vi "GUI_Cameras_GRID.vi"() -> ()   [LabVIEW 2011]
uses:
  <vilib>/Utility/miscctls.llb/LVRectTypeDef.ctl
  <vilib>/vision/NI_Vision_Development_Module.lvlib
panel:
  in  "Tab Control":T1(tab)
  in  "analysis":bool
  out "MaxCounts":dbl(slide) scale=0.0..256.0
  in  "triggerdelay":dbl
  in  "trigger":bool
  in  "save":bool
  in  "exposure":dbl=0.52 caption="Exposure"
  in  "gain":dbl
  in  "shotnumber":i32=354
  out "Centroid":cluster{"X Centroid":sgl, "Y Centroid":sgl} {"Y Centroid" format="%.2f"; "X Centroid" format="%.2f"}
  out "Mean Value":sgl format="%.2f"
  out "Mean Value 2":sgl(graph)
  out "histogram":T2(graph)
  out "lineout":cluster{"x0":sgl, "dx":sgl, "Pixels Line":sgl[]}(graph)
  out "analysis error":errorcluster
  out "Zoom changed":bool
  out "Zoom old":cluster{"X":sgl, "Y":sgl}
  out "ratio(h)":bool=TRUE
  out "fixsize":bool
  out "Change Ratio":cluster{"X":sgl, "Y":sgl}={"X"=1.6671598, "Y"=0.6151203}
  out "old Panel Bounds":T3={"Left"=105, "Top"=80, "Right"=781, "Bottom"=662}
  out "error (h)":bool
  in  "Main Tap":enum32{"IMAQ", "Network", "Internal", "Array"}(tab)
  out "Image (IMAQ)":T4(plugin-control)
  out "local Port":u16=65401
  out "Remote Host":string="192.168.10.157"
  out "port or service name":u16=65400
  in  "timeout ms (slow resp)":i32=500
  in  "reset":bool
  out "All Devices (h)":string[](array[string])
  out "centroidy":dbl
  out "fast ID (h)":refnum<k16>
  out "slow ID (h)":refnum<k16>
  out "error out":errorcluster
  out "connections (hidden)":variant[](array[variant])=[variant(refnum<k16> refnum), variant(refnum<k16> refnum)]
  in  "time to wait (main loop)":i32=200
  in  "time to wait (TCP)":i32=10
  out "Data String":string="exposure,0.520000\r\ntrigger,off\r\nsave,off\r\ngain,0.000000\r\n"
  in  "send":bool
  in  "localsavingpath":path
  out "centroidy":dbl
  out "Image (array)":u8[][](graph)
  out "Device Name (h)":string="FakeCam1"
  out "stop":bool
  out "error message":string
  out "image connection":bool
  out "data connection ok":bool
  # "Data"
  # "Image"
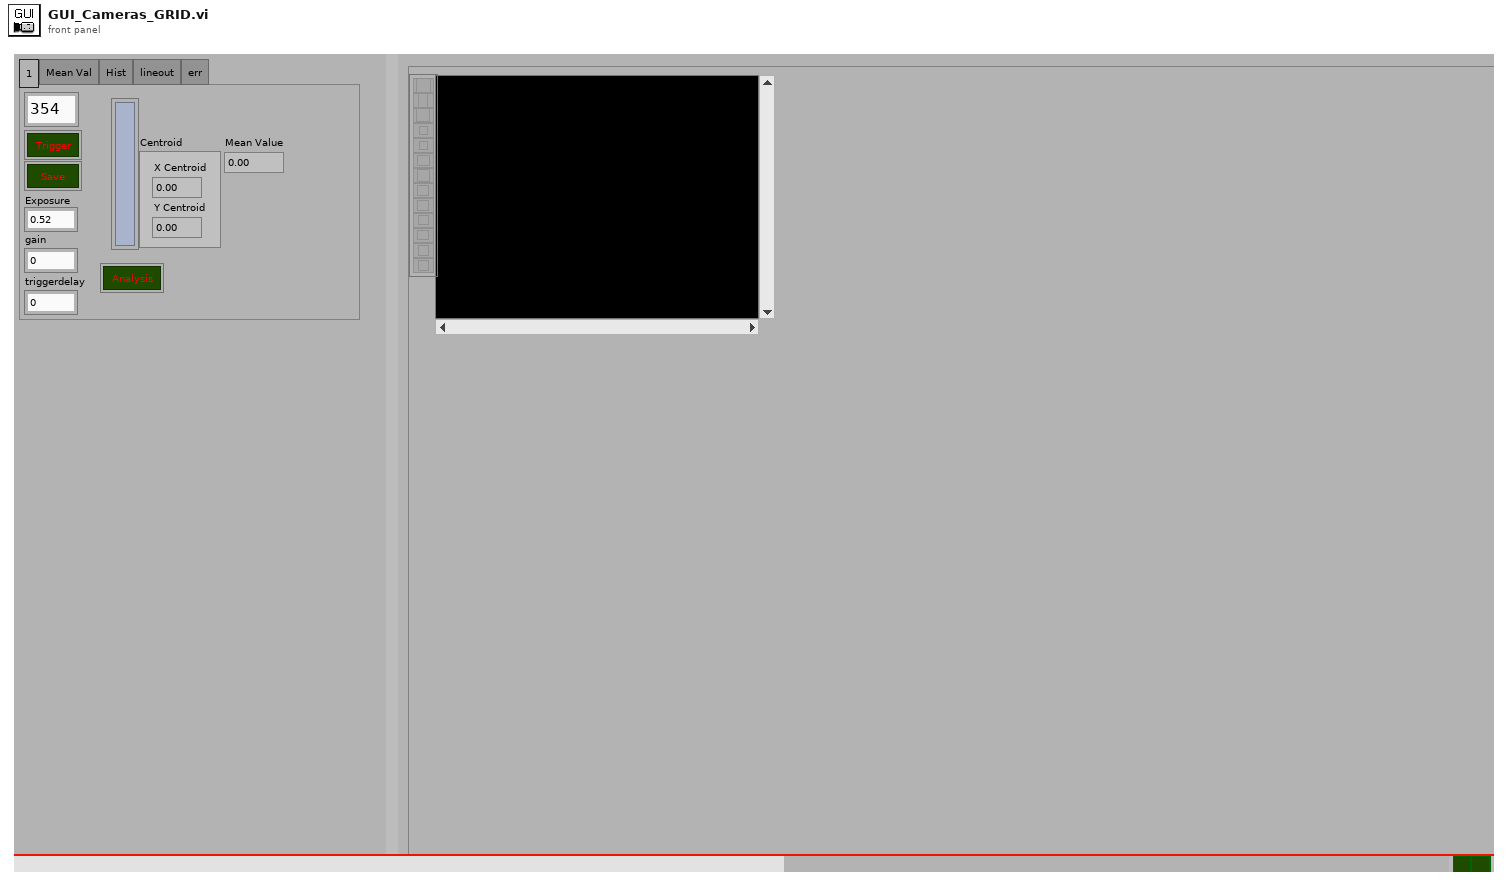
[diagram p1: front panel]
types:
  T1 = enum32{"1", "Mean Val", "Hist", "lineout", "err"}
  T2 = cluster{"Starting Value":sgl, "Incremental Value":sgl, "Histogram":u32[]}
  T3 = typedef "LVRectTypeDef.ctl" = cluster{"Left":i16, "Top":i16, "Right":i16, "Bottom":i16}
  T4 = typedef "IMAQ Image.ctl" = refnum<image>
  T5 = enum16{"Grayscale", "Binary", "Gradient", "Rainbow", "Temperature", "User Defined"}
  T6 = typedef "Image Type" = u32
  T7 = cluster{"Global Rectangle":i32[], "Contours":cluster{"Contour Type":u32, "ROI Type":u32, "Points":i32[]}[]}
  T8 = typedef "IMAQ Line" = cluster{"Start X":i32, "Start Y":i32, "End X":i32, "End Y":i32}
  T9 = typedef "ROI Descriptor" = cluster{"Global Rectangle":i32[], "Contours":cluster{"ID":enum32{"External", "Internal"}, "Type":u32, "Coordinates":i32[]}[]}
  T10 = typedef "LVBoundsTypeDef.ctl" = cluster{"Width":u32, "Height":u32}
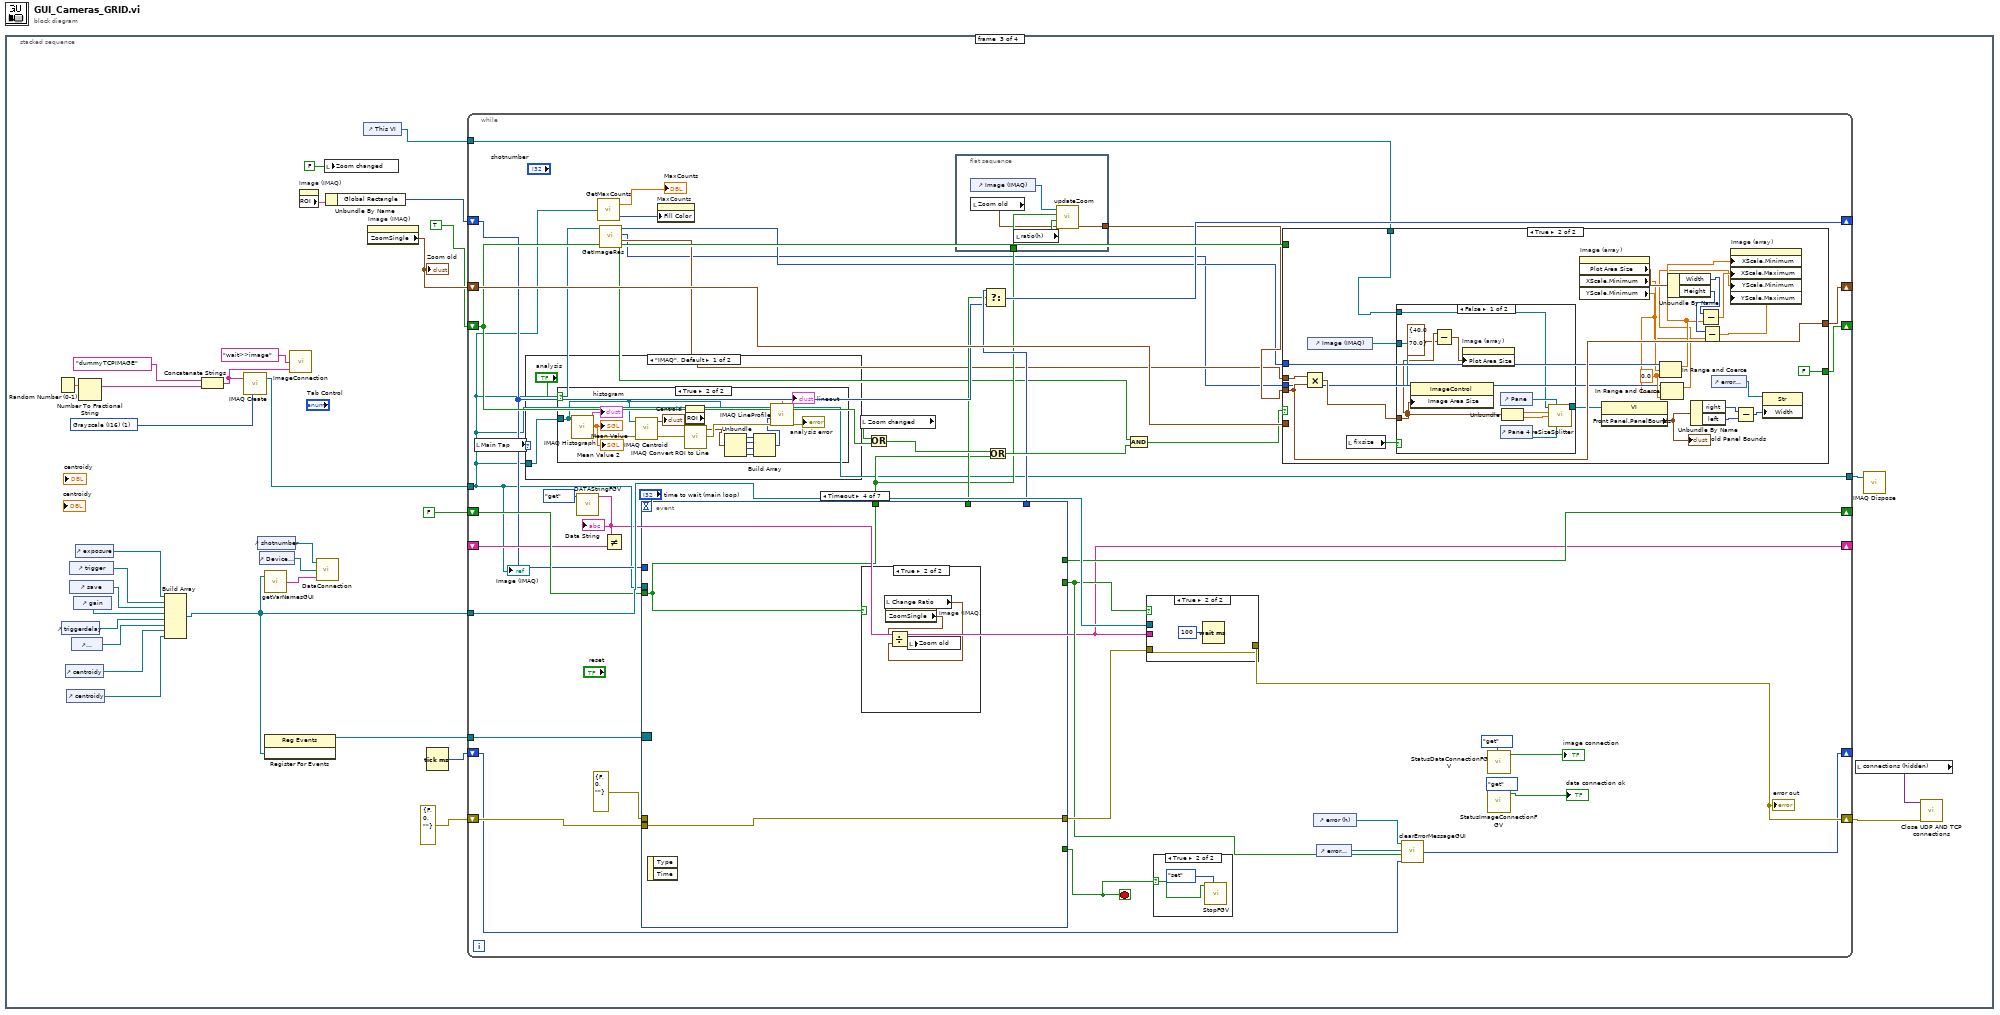
[diagram p0: block diagram]
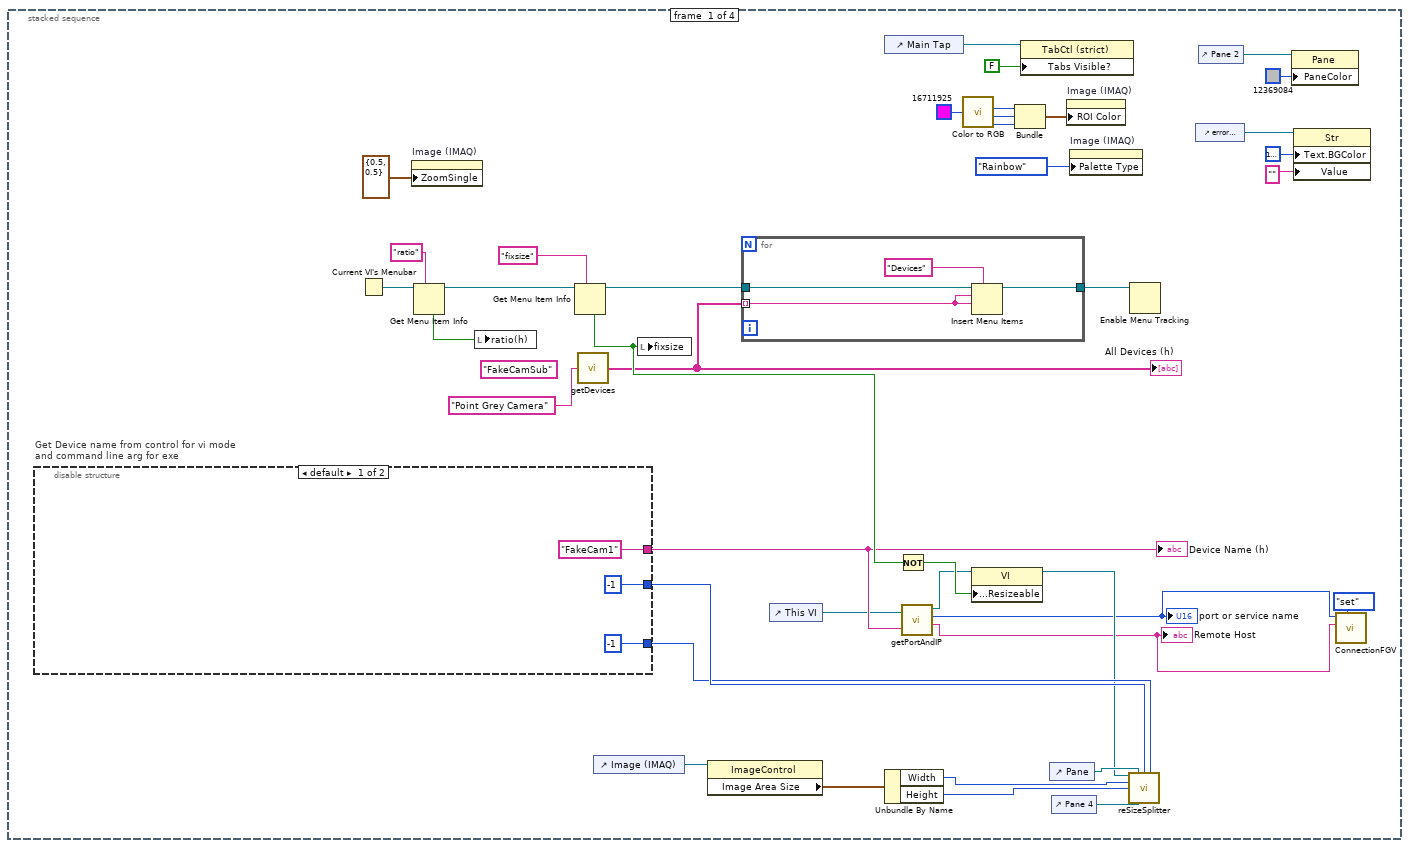
[diagram p2: hidden frame]
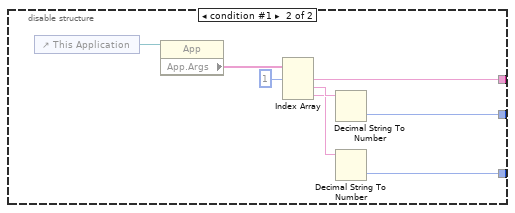
[diagram p3: hidden frame]
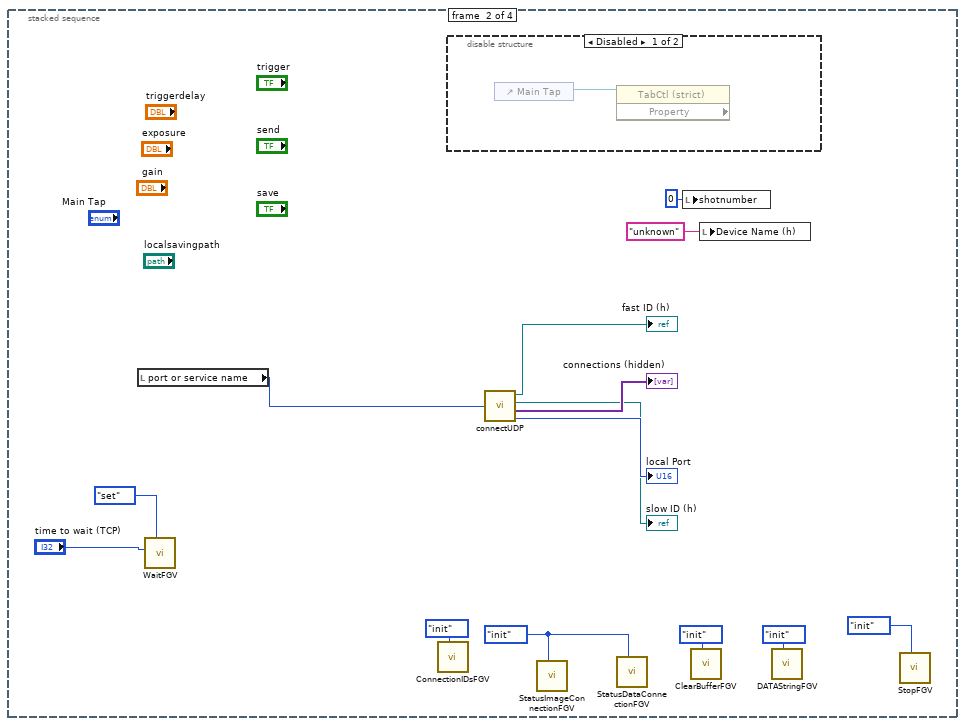
[diagram p4: hidden frame]
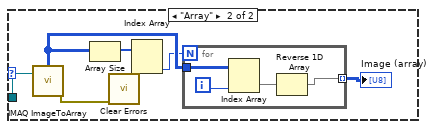
[diagram p8: hidden frame]
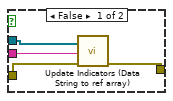
[diagram p11: hidden frame]
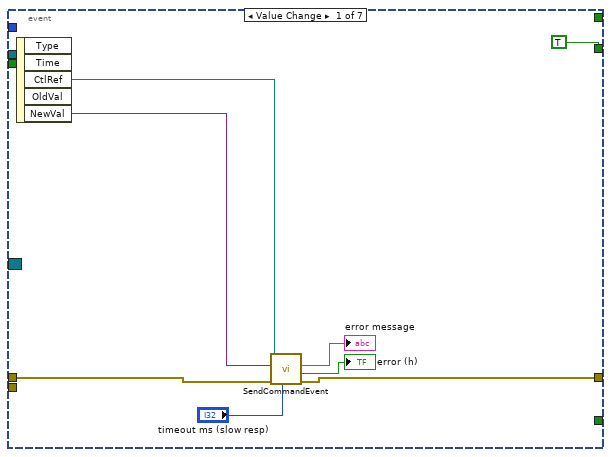
[diagram p12: hidden frame]
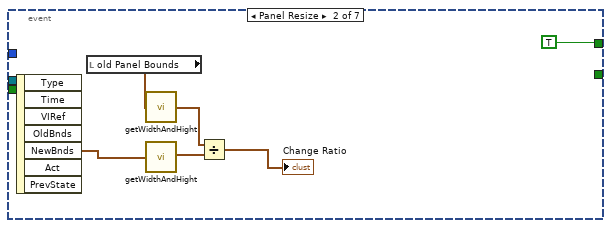
[diagram p13: hidden frame]
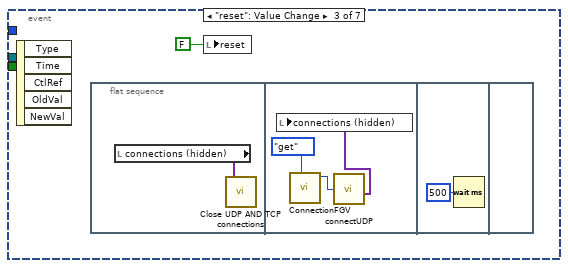
[diagram p14: hidden frame]
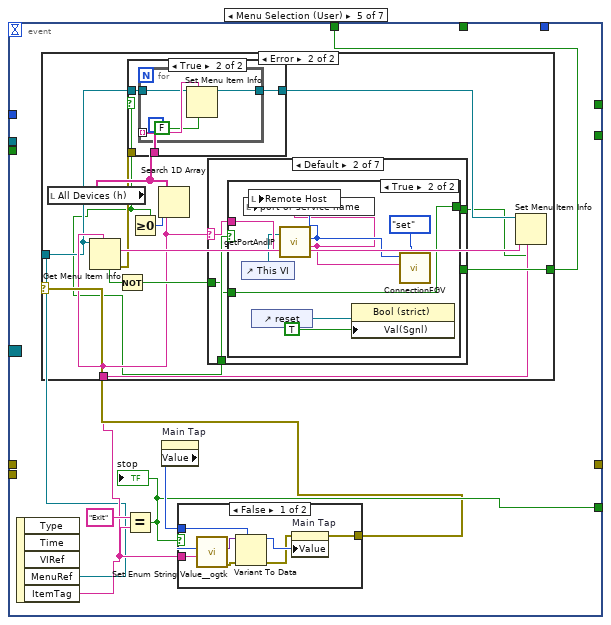
[diagram p16: hidden frame]
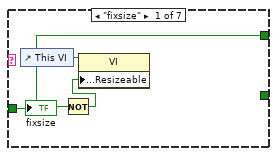
[diagram p19: hidden frame]
diagram:
  n1 = stacked-sequence {
    frame #0 {
      (unwired) "FakeCamSub" ("Device Class")
      n2 = disable-structure "Get Device name from control for vi mode\nand command line arg for exe" shown="default" {
        disable-tunnel: ["FakeCam1" ("Device Name for vi mode") w52] -> w14
        disable-tunnel: [i16 -1 ("left") w49] -> w27
        disable-tunnel: [i16 -1 ("left") w48] -> w26
        frame condition #0 (active) {
        }
        frame condition #1 {
          n3 = control-ref of="This Application"() -> (w55:refnum<vi>)
          n4 = property class="App"(reference=w55) -> ("App.Args"=w54:string[])  [unwired: 1 in, 2 out]
          n5 = Index Array(array=w54, index #1=1 ("index")) -> (element #1=w52:string, element #2=w51:string, element #3=w50:string)  [unwired: 2 in]
          n6 = Decimal String To Number(string=w51) -> (number=w49:i32)  [unwired: 2 in, 1 out]
          n7 = Decimal String To Number(string=w50) -> (number=w48:i32)  [unwired: 2 in, 1 out]
        }
      }
      "Device Name (h)" <- w14
      n8 = Current VI's Menubar() -> (w31:refnum<k9>)
      n9 = property on="Image (IMAQ)" class="ImageControl"("ZoomSingle"=cluster{"X":sgl, "Y":sgl} {"X"=0.5, "Y"=0.5} ("ZoomSingle:All Elements")) -> ()  [unwired: 2 in, 2 out]
      n10 = Get Menu Item Info(7:"ratio" ("item tag"), 11:w31) -> (3:w29:refnum<k9>, 4:w30:bool)  [unwired: 1 in, 5 out]
      n11 = local write "ratio(h)"(w30) -> ()
      n12 = Get Menu Item Info(7:"fixsize" ("item tag"), 11:w29) -> (3:w17:refnum<k9>, 4:w24:bool)  [unwired: 1 in, 5 out]
      n13 = call "getDevices.vi"("Device Class"="Point Grey Camera") -> ("All Devices"=w15:string[])
      "All Devices (h)" <- w15
      n14 = control-ref of="Image (IMAQ)"() -> (w38:refnum<vi>)
      n15 = local write "fixsize"(w24) -> ()
      n16 = property class="ImageControl"(reference=w38) -> ("Image Area Size"=w37:cluster{"Width":u32, "Height":u32})  [unwired: 1 in, 2 out]
      n17 = for {
        tunnel: w17 -> [w44]
        tunnel: [w43] -> w16
        tunnel: w15 -> [w41] mode=indexing
        n18 = Insert Menu Items(5:"Devices" ("menu tag"), 7:w41, 8:w41, 9:w44) -> (3:w43:refnum<k9>)  [unwired: 2 in, 2 out]
      }
      n19 = control-ref of="This VI"() -> (w13:refnum<vi>)
      n20 = control-ref of="Main Tap"() -> (w40:refnum<vi>)
      n21 = Unbundle By Name(w37) -> ("Width"=w36:u32, "Height"=w35:u32)
      n22 = Not(x=w24) -> (.not. x?=w25:bool)
      n23 = call "getPortAndIP.vi"("This Vi"=w13, "Device Name"=w14) -> ("reference out"=w12:refnum<vi>, "port or service name"=w3:u16, "Remote Host"=w2:string)  [unwired: 1 in]
      "port or service name" <- w3
      "Remote Host" <- w2
      n24 = call <vilib>:"Color to RGB.vi"("Color"=u32 16711925) -> ("R"=w9:u8, "G"=w8:u8, "B"=w7:u8)  [unwired: 1 out]
      n25 = property class="VI"(reference=w12, "Front Panel.Resizeable"=w25) -> (reference out=w5:refnum<vi>)  [unwired: 1 in, 1 out]
      n26 = Bundle("R"=w9, "G"=w8, "B"=w7) -> (w6:cluster{"R":u8, "G":u8, "B":u8})  [unwired: 1 in]
      n27 = property class="TabCtl (strict)"(reference=w40, "Tabs Visible?"=FALSE) -> ()  [unwired: 1 in, 2 out]
      n28 = control-ref of="Pane"() -> (w34:refnum<vi>)
      n29 = control-ref of="Pane 4"() -> (w23:refnum<vi>)
      n30 = property on="Image (IMAQ)" class="ImageControl"("ROI Color"=w6) -> ()  [unwired: 2 in, 2 out]
      n31 = property on="Image (IMAQ)" class="ImageControl"("Palette Type"=T5."Rainbow" ("Palette:Palette Type")) -> ()  [unwired: 2 in, 2 out]
      n32 = call "reSizeSplitter.vi"("this vi"=w5, "pane"=w34, "left"=w27, "top"=w26, "Width"=w36, "Height"=w35, "pane2"=w23) -> ()  [unwired: 8 in, 1 out]
      n33 = Enable Menu Tracking(4:w16) -> ()  [unwired: 2 in, 2 out]
      n34 = control-ref of="error message"() -> (w21:refnum<vi>)
      n35 = control-ref of="Pane 2"() -> (w19:refnum<vi>)
      n36 = property class="Pane"(reference=w19, "PaneColor"=u32 12369084) -> ()  [unwired: 1 in, 2 out]
      n37 = property class="Str"(reference=w21, "Text.BGColor"=u32 16777238, "Value"="") -> ()  [unwired: 1 in, 2 out]
      n38 = call "ConnectionFGV.vi"("command"=enum16{"get", "set", "init"}."set", "Remote Host in"=w2, "port or service name in"=w3) -> ()  [unwired: 7 in, 2 out]
    }
    frame #1 {
      w65 = enum16{"get", "set", "init"}."init" ("Command")
      n39 = local read "port or service name"() -> (w67:u16)
      n40 = call "WaitFGV.vi"("Command"=enum16{"get", "set", "init"}."set", "milliseconds to wait"="time to wait (TCP)") -> ()  [unwired: 9 in, 1 out]
      n41 = call "ConnectionIDsFGV.vi"("Command"=enum16{"add", "get", "init"}."init") -> ()  [unwired: 10 in, 1 out]
      n42 = disable-structure shown="Disabled" {
        frame Disabled {
          n43 = control-ref of="Main Tap"() -> (w70:refnum<vi>)
          n44 = property class="TabCtl (strict)" props=[](reference=w70) -> ()  [unwired: 1 in, 3 out]
        }
        frame Enabled {
        }
      }
      n45 = call "connectUDP.vi"("port or service name"=w67) -> ("fast ID (h)"=→"fast ID (h)":refnum<k16>, "slow ID (h)"=→"slow ID (h)":refnum<k16>, "connections (hidden)"=→"connections (hidden)":variant[], "local Port"=→"local Port":u16)
      n46 = call "StatusImageConnectionFGV.vi"("Command"=w65) -> ()  [unwired: 10 in, 1 out]
      n47 = call "StatusDataConnectionFGV.vi"("Command"=w65) -> ()  [unwired: 10 in, 1 out]
      n48 = local write "shotnumber"(0 ("shotnumber")) -> ()
      n49 = call "ClearBufferFGV.vi"("Command"=enum16{"set", "get", "init"}."init") -> ()  [unwired: 10 in, 1 out]
      n50 = local write "Device Name (h)"("unknown" ("Device Name")) -> ()
      n51 = call "DATAStringFGV.vi"("Command"=enum16{"get", "set", "init"}."init") -> ()  [unwired: 10 in, 1 out]
      n52 = call "StopFGV.vi"("Command"=enum16{"set", "get", "init"}."init") -> ()  [unwired: 10 in, 1 out]
    }
    frame #2 {
      w100 = T6 1 items=["Grayscale (U8)", "Grayscale (I16)", "Grayscale (SGL)", "Complex (CSG)", "RGB (U32)", "HSL (U32)", "RGB (U64)", "Grayscale (U16)"] ("Image Type")
      n53 = Random Number (0-1)() -> (number: 0 to 1=w97:dbl)
      n54 = control-ref of="triggerdelay"() -> (w87:refnum<vi>)
      n55 = control-ref of="centroidy"() -> (w81:refnum<vi>)
      n56 = control-ref of="centroidy"() -> (w74:refnum<vi>)
      n57 = control-ref of="trigger"() -> (w91:refnum<vi>)
      n58 = control-ref of="save"() -> (w89:refnum<vi>)
      n59 = control-ref of="localsavingpath"() -> (w82:refnum<vi>)
      n60 = control-ref of="gain"() -> (w88:refnum<vi>)
      n61 = control-ref of="exposure"() -> (w90:refnum<vi>)
      n62 = Number To Fractional String(number=w97) -> (F-format string=w96:string)  [unwired: 3 in]
      n63 = Build Array(w90, w91, w89, w88, w87, w82, w81, w74) -> (w72:refnum<vi>[])
      n64 = Concatenate Strings("dummyTCPIMAGE" ("Image Name"), w96) -> (w94:string)
      n65 = call "IMAQ Create"("Image Name"=w94, "Image Type"=w100) -> ("New Image"=w99:T4)  [unwired: 3 in, 1 out]
      n66 = control-ref of="shotnumber"() -> (w76:refnum<vi>)
      n67 = control-ref of="Device Name (h)"() -> (w75:refnum<vi>)
      n68 = call "getVarNamesGUI.vi"("Array"=w72) -> ("String"=w71:string)  [unwired: 1 in]
      n69 = register-events(w72) -> (reference out=w73:refnum<event-registration>)  [unwired: 2 in, 1 out]
      n70 = call "ImageConnection.vi"("Image Name"=w94, "Image Subscriber list"="wait>>image") -> ()  [unwired: 2 in]
      n71 = property on="Image (IMAQ)" class="ImageControl"() -> ("ROI"=w80:T7)  [unwired: 2 in, 2 out]
      n72 = call "DataConnection.vi"("Subscriber list"=w71, "Device Name (h)"=w75, "shotnumber"=w76) -> ()
      n73 = local write "Zoom changed"(FALSE ("Zoom changed")) -> ()
      n74 = Unbundle By Name(w80) -> ("Global Rectangle"=w79:i32[])
      n75 = control-ref of="This VI"() -> (w78:refnum<vi>)
      n76 = property on="Image (IMAQ)" class="ImageControl"() -> ("ZoomSingle"=w86:cluster{"X":sgl, "Y":sgl})  [unwired: 2 in, 2 out]
      "Zoom old" <- w86
      n77 = Tick Count (ms)() -> (millisecond timer value=w83:u32)
      n78 = while {
        shift-right: [w142] -> w98
        shift-left: errorcluster {"status"=FALSE, "code"=0, "source"=""} ("error out") -> [w144]
        tunnel: w99 -> [w116]
        tunnel: [w116] -> w101
        tunnel: w72 -> [w146]
        shift-right: [w141] -> _
        shift-left: w86 -> [w140]
        shift-right: [w138] -> _
        shift-left: FALSE -> [w139]
        shift-right: [w137] -> _
        shift-left: TRUE -> [w136]
        shift-right: [w132] -> _
        shift-left: w83 -> [w131]
        shift-right: [w105] -> _
        shift-left: _ -> [w129]
        shift-right: [w125] -> _
        shift-left: w79 -> [w124]
        tunnel: w78 -> [w122]
        tunnel: w73 -> [w103]
        stop <- w106 stop-if-true
        n79 = local read "Main Tap"() -> (w127:enum32{"IMAQ", "Network", "Internal", "Array"})
        n80 = case shown="\"IMAQ\", Default" w127 {
          tunnel: w116 -> [w156 w177]
          frame "IMAQ", Default {
            n81 = case shown="True" "analysis" {
              tunnel: w156 -> [_ w167]
              frame False {
              }
              frame True {
                n82 = call "IMAQ Histograph"("Image"=w167) -> ("error out"=w169:errorcluster, "Mean Value"=→"Mean Value" →"Mean Value 2":sgl, "Histogram Graph"=→"histogram":T2)  [unwired: 7 in, 1 out]
                n83 = call "IMAQ Centroid"("error in (no error)"=w169, "Image"=w167) -> ("error out"=w166:errorcluster, "Centroid"=→"Centroid":cluster{"X Centroid":sgl, "Y Centroid":sgl})  [unwired: 2 in]
                n84 = property on="Image (IMAQ)" class="ImageControl"() -> ("ROI"=w163:T7)  [unwired: 2 in, 2 out]
                n85 = call "IMAQ Convert ROI to Line"("ROI Descriptor"=w163) -> ("Line"=w162:T8)  [unwired: 8 in, 1 out]
                n86 = Unbundle(w162) -> ("Start X"=w161:i32, "Start Y"=w160:i32, "End X"=w159:i32, "End Y"=w158:i32)
                n87 = Build Array(w161, w160, w159, w158) -> (w157:i32[])
                n88 = call "IMAQ LineProfile"("error in (no error)"=w166, "Line Coordinates"=w157, "Image"=w167) -> ("error out"=→"analysis error":errorcluster, "Line Graph"=→"lineout":cluster{"x0":sgl, "dx":sgl, "Pixels Line":sgl[]})  [unwired: 2 in, 2 out]
              }
            }
          }
          frame "Array" {
            n89 = call "IMAQ ImageToArray"("Image"=w177) -> ("error out"=w176:errorcluster, "Image Pixels (U8)"=w173:u8[][])  [unwired: 3 in, 3 out]
            n90 = Array Size(array=w173) -> (size(s)=w175:i32[])
            n91 = call <vilib>:"Clear Errors.vi"("error in (no error)"=w176) -> ()  [unwired: 6 in, 1 out]
            n92 = Index Array(array=w175) -> (element #2=w172:i32)  [unwired: 2 in, 1 out]
            n93 = for {
              N: w172 -> [_]
              tunnel: w173 -> [w181]
              tunnel: [w179] -> w174 mode=indexing
              i -> [w178]
              n94 = Index Array(array=w181, index (col)=w178) -> (element=w180:u8[])  [unwired: 1 in]
              n95 = Reverse 1D Array(array=w180) -> (reversed array=w179:u8[])
            }
            "Image (array)" <- w174
          }
        }
        n96 = call "DATAStringFGV.vi"("Command"=enum16{"get", "set", "init"}."get") -> ("Data String out"=w105:string)  [unwired: 10 in]
        "Data String" <- w105
        n97 = call "GetMaxCounts.vi"("New Image"=w116) -> ("Maximal Value"=→"MaxCounts":sgl, "Color"=w118:u32)
        n98 = call "GetImageRes.vi"("Image"=w116) -> ("valid Image"=w114:bool, "Image Area:Size:All Elements"=w115:cluster{"Width":u32, "Height":u32}, "Y Resolution"=w112:i32, "X Resolution"=w113:i32)  [unwired: 7 in]
        n99 = Not Equal?(x=w105, y=w129) -> ()  [unwired: 1 out]
        n100 = event shown="[3] Timeout" {
          selector: w103 -> [_ _ _ _ _ _ _]
          dyn-events: _ -> [_ _ _ _ _ _ _]
          timeout: "time to wait (main loop)" -> [_ _ _ _ _ _ _]
          tunnel: [w231 _ _ w247 _ _ _] -> w143
          tunnel: errorcluster {"status"=FALSE, "code"=0, "source"=""} ("error out") -> [w233 _ _ _ _ _ _]
          tunnel: w144 -> [_ _ _ w247 _ _ _]
          tunnel: [TRUE _ _ _ _ _ _] -> w128
          tunnel: [_ _ _ _ w255 _ _] -> w106
          tunnel: [_ _ _ w246 w252 _ _] -> w121
          tunnel: w139 -> [_ _ _ w246 _ _ _]
          tunnel: [_ TRUE _ _ _ _ _] -> w138
          tunnel: [_ _ _ _ _ _ w333] -> w126
          tunnel: w124 -> [_ _ _ _ _ _ w334]
          tunnel: [_ _ _ _ _ _ w327] -> w123
          tunnel: w116 -> [_ _ _ _ _ _ w336]
          event Value Change {
            n101 = event-data() -> ("CtlRef"=w228:refnum<vi>, "NewVal"=w227:variant)  [unwired: 1 in, 3 out]
            n102 = call "SendCommandEvent.vi"("timeout ms (slow resp)"="timeout ms (slow resp)", "error out 2"=w233, "NewVal"=w227, "CtlRef"=w228) -> ("error out"=w231:errorcluster, "error (h)"=→"error (h)":bool, "error message"=→"error message":string)  [unwired: 4 in, 1 out]
          }
          event Panel Resize {
            n103 = event-data() -> ("NewBnds"=w239:T3)  [unwired: 1 in, 6 out]
            n104 = local read "old Panel Bounds"() -> (w237:T3)
            n105 = call "getWidthAndHight.vi"("OldBnds"=w237) -> ("output cluster"=w236:cluster{"X":sgl, "Y":sgl})
            n106 = call "getWidthAndHight.vi"("OldBnds"=w239) -> ("output cluster"=w235:cluster{"X":sgl, "Y":sgl})
            n107 = Divide(x=w236, y=w235) -> (x/y=→"Change Ratio":cluster{"X":sgl, "Y":sgl})
          }
          event "reset": Value Change {
            n108 = event-data() -> ()  [unwired: 1 in, 5 out]
            n109 = flat-sequence {
              frame #0 {
                n110 = local read "connections (hidden)"() -> (w241:variant[])
                n111 = call "Close UDP AND TCP connections.vi"("appended array"=w241) -> ()  [unwired: 7 in]
              }
              frame #1 {
                n112 = call "ConnectionFGV.vi"("command"=enum16{"get", "set", "init"}."get") -> ("port or service name out"=w243:u16)  [unwired: 9 in, 1 out]
                n113 = call "connectUDP.vi"("port or service name"=w243) -> ("connections (hidden)"=w242:variant[])  [unwired: 3 out]
                n114 = local write "connections (hidden)"(w242) -> ()
              }
              frame #2 {
                n115 = Wait (ms)(milliseconds to wait=u32 500) -> ()  [unwired: 1 out]
              }
              frame #3 {
              }
            }
            n116 = local write "reset"(FALSE ("reset")) -> ()
          }
          event Timeout {
            n117 = event-data() -> ()  [unwired: 1 in, 2 out]
            n118 = case shown="True" w246 {
              frame False {
              }
              frame True {
                n119 = local read "Change Ratio"() -> (w249:cluster{"X":sgl, "Y":sgl})
                n120 = property on="Image (IMAQ)" class="ImageControl"() -> ("ZoomSingle"=w250:cluster{"X":sgl, "Y":sgl})  [unwired: 2 in, 2 out]
                n121 = Divide(x=w250, y=w249) -> (x/y=w248:cluster{"X":sgl, "Y":sgl})
                n122 = local write "Zoom old"(w248) -> ()
              }
            }
          }
          event Menu Selection (User) {
            n123 = event-data() -> ("MenuRef"=w251:refnum<k9>, "ItemTag"=w253:string)  [unwired: 1 in, 3 out]
            n124 = Equal?(x="Exit", y=w253) -> (x = y?=w255:bool)
            "stop" <- w255
            n125 = property on="Main Tap" class="TabCtl (strict)"() -> ("Value"=w257:enum32{"IMAQ", "Network", "Internal", "Array"})  [unwired: 2 in, 2 out]
            n126 = case shown="False" w255 {
              tunnel: w257 -> [w316 _]
              tunnel: w253 -> [w315 _]
              tunnel: [w312 errorcluster {"status"=FALSE, "code"=0, "source"=""} ("error out")] -> w254
              frame False {
                n127 = call <userlib>:"Set Enum String Value__ogtk.vi"("String Value"=w315, "Default Enum Value"=w316) -> ("error out"=w314:errorcluster, "Enum"=w318:variant)  [unwired: 8 in]
                n128 = Variant To Data(error in=w314, type=w316, Variant=w318) -> (data=w317:enum32{"IMAQ", "Network", "Internal", "Array"}, error out=w313:errorcluster)
                n129 = property on="Main Tap" class="TabCtl (strict)"(error in=w313, "Value"=w317) -> (error out=w312:errorcluster)  [unwired: 1 in, 1 out]
              }
              frame True {
              }
            }
            n130 = case shown="Error" w254 {
              tunnel: w251 -> [_ w261]
              tunnel: w253 -> [_ w265]
              tunnel: [_ w266] -> w252
              frame No Error {
              }
              frame Error {
                n131 = local read "All Devices (h)"() -> (w263:string[])
                n132 = Get Menu Item Info(7:w265, 11:w261) -> (0:w262:errorcluster, 2:w268:string, 4:w269:bool)  [unwired: 1 in, 4 out]
                n133 = Not(x=w269) -> (.not. x?=w267:bool)
                n134 = Search 1D Array(1D array=w263, element=w265) -> (index of element=w264:i32)  [unwired: 1 in]
                n135 = Greater Or Equal To 0?(x=w264) -> (x >= 0?=w260:bool)
                n136 = case shown="True" w260 {
                  tunnel: w263 -> [_ w273]
                  tunnel: w262 -> [_ _]
                  tunnel: w261 -> [w270 w272]
                  tunnel: [w270 w271] -> w259
                  frame False {
                  }
                  frame True {
                    n137 = for {
                      tunnel: w273 -> [w277] mode=indexing
                      tunnel: w272 -> [w275]
                      tunnel: [w274] -> w271
                      n138 = Set Menu Item Info(6:FALSE ("checked"), 7:w277, 11:w275) -> (3:w274:refnum<k9>)  [unwired: 4 in, 1 out]
                    }
                  }
                }
                n139 = case shown="Default" w265 {
                  selector: w265 -> [_ w283 _ _ w304 _ _]
                  tunnel: w267 -> [w278 w281 w294 _ _ _ w309]
                  tunnel: [_ _ TRUE _ _ _ _] -> w266
                  tunnel: w260 -> [_ w284 _ _ _ _ _]
                  tunnel: [w278 w282 w294 _ _ _ w309] -> w258
                  frame "fixsize" {
                    n140 = control-ref of="This VI"() -> (w280:refnum<vi>)
                    n141 = Not(x=w278) -> (.not. x?=w279:bool)
                    n142 = property class="VI"(reference=w280, "Front Panel.Resizeable"=w279) -> ()  [unwired: 1 in, 2 out]
                    "fixsize" <- w278
                  }
                  frame Default {
                    n143 = case shown="True" w284 {
                      tunnel: w283 -> [_ w292]
                      tunnel: [_ w288] -> w282
                      tunnel: w281 -> [_ w288]
                      frame False {
                      }
                      frame True {
                        n144 = control-ref of="This VI"() -> (w291:refnum<vi>)
                        n145 = control-ref of="reset"() -> (w290:refnum<vi>)
                        n146 = call "getPortAndIP.vi"("This Vi"=w291, "Device Name"=w292) -> ("port or service name"=w286:u16, "Remote Host"=w285:string)  [unwired: 1 in, 1 out]
                        n147 = local write "port or service name"(w286) -> ()
                        n148 = local write "Remote Host"(w285) -> ()
                        n149 = property class="Bool (strict)"(reference=w290, "Val(Sgnl)"=TRUE ("Value (Signaling)")) -> ()  [unwired: 1 in, 2 out]
                        n150 = call "ConnectionFGV.vi"("command"=enum16{"get", "set", "init"}."set", "Remote Host in"=w285, "port or service name in"=w286) -> ()  [unwired: 7 in, 2 out]
                      }
                    }
                  }
                  frame "ratio" {
                    n151 = property on="Image (IMAQ)" class="ImageControl"() -> ("ZoomSingle"=w293:cluster{"X":sgl, "Y":sgl})  [unwired: 2 in, 2 out]
                    n152 = local write "Zoom old"(w293) -> ()
                    "ratio(h)" <- w294
                  }
                  frame "Local Saving Path" {
                    n153 = control-ref of="localsavingpath"() -> (w296:refnum<vi>)
                    n154 = property class="Path"(reference=w296) -> (reference out=w299:refnum<vi>, "Value"=w300:path)  [unwired: 1 in, 1 out]
                    n155 = call "changePath.vi"("Local Saving in (h)"=w300) -> ("change (h)"=w298:bool, "Local Saving out (h)"=w297:path)  [unwired: 9 in]
                    n156 = case shown="True" w298 {
                      tunnel: w299 -> [_ w302]
                      tunnel: w297 -> [_ w301]
                      frame False {
                      }
                      frame True {
                        n157 = property class="Path"(reference=w302, "Val(Sgnl)"=w301) -> ()  [unwired: 1 in, 2 out]
                      }
                    }
                  }
                  frame "Binary", "Gradient", "Grayscale", "Rainbow", "Temperature" {
                    n158 = Scan From String(input string=w304, default 1=T5."Grayscale" ("Palette:Palette Type")) -> (output 1=w303:T5)  [unwired: 3 in, 3 out]
                    n159 = property on="Image (IMAQ)" class="ImageControl"("Palette Type"=w303) -> ()  [unwired: 2 in, 2 out]
                  }
                  frame "reset" {
                    n160 = control-ref of="reset"() -> (w307:refnum<vi>)
                    n161 = property class="Bool (strict)"(reference=w307, "Val(Sgnl)"=TRUE ("Value (Signaling)")) -> ()  [unwired: 1 in, 2 out]
                  }
                  frame "clear" {
                    n162 = control-ref of="reset"() -> (w311:refnum<vi>)
                    n163 = call "ClearBufferFGV.vi"("Command"=enum16{"set", "get", "init"}."set", "clear buffer"=w309) -> ()  [unwired: 9 in, 1 out]
                    n164 = property class="Bool (strict)"(reference=w311, "Val(Sgnl)"=TRUE ("Value (Signaling)")) -> ()  [unwired: 1 in, 2 out]
                  }
                }
                n165 = Set Menu Item Info(6:w258, 7:w265, 10:w268, 11:w259) -> ()  [unwired: 3 in, 2 out]
              }
            }
          }
          event "time to wait (TCP)": Value Change {
            n166 = event-data() -> ("NewVal"=w321:i32)  [unwired: 1 in, 4 out]
            n167 = call "WaitFGV.vi"("Command"=enum16{"get", "set", "init"}."set", "milliseconds to wait"=w321) -> ()  [unwired: 9 in, 1 out]
          }
          event "Image (IMAQ)": Mouse Up {
            n168 = event-data() -> ()  [unwired: 1 in, 5 out]
            n169 = property on="Image (IMAQ)" class="ImageControl"() -> ("ROI"=w335:T7)  [unwired: 2 in, 2 out]
            n170 = Unbundle By Name(w335) -> ("Global Rectangle"=w333:i32[])
            n171 = Not Equal?(x=w334, y=w333) -> (x != y?=w337:bool[])
            n172 = property on="Image (IMAQ)" class="ImageControl"() -> ("ZoomSingle"=w322:cluster{"X":sgl, "Y":sgl})  [unwired: 2 in, 2 out]
            n173 = local read "Zoom old"() -> (w324:cluster{"X":sgl, "Y":sgl})
            n174 = Empty Array?(array=w334) -> (empty?=w330:bool)
            n175 = Empty Array?(array=w333) -> (empty?=w332:bool)
            n176 = Or Array Elements(Boolean array=w337) -> (logical OR=w328:bool)
            n177 = Not(x=w332) -> (.not. x?=w331:bool)
            n178 = And(x=w330, y=w331) -> (x .and. y?=w329:bool)
            n179 = Unbundle By Name(w322) -> ("X"=w325:sgl)
            n180 = Unbundle By Name(w324) -> ("X"=w326:sgl)
            n181 = Not Equal?(x=w325, y=w326) -> (x != y?=w323:bool)
            "Zoom changed" <- w323
            n182 = Or(x=w328, y=w329) -> (x .or. y?=w327:bool)
            n183 = case shown="True" w327 {
              tunnel: w336 -> [_ _]
              tunnel: w335 -> [_ w340]
              frame False {
              }
              frame True {
                n184 = call "ROI thickener.vi"("ROI Descriptor in"=w340) -> ("ROI Descriptor out"=w339:T9)  [unwired: 1 in, 1 out]
                n185 = property on="Image (IMAQ)" class="ImageControl"("ROI"=w339) -> ()  [unwired: 2 in, 2 out]
              }
            }
            n186 = case shown="True" w323 {
              tunnel: w322 -> [_ w338]
              frame False {
              }
              frame True {
                n187 = local write "Zoom old"(w338) -> ()
              }
            }
          }
        }
        n188 = property on="MaxCounts" class="Slide (strict)"("Fill Color"=w118) -> ()  [unwired: 2 in, 2 out]
        n189 = local read "Zoom changed"() -> (w117:bool)
        n190 = Or(x=w117, y=w136) -> (x .or. y?=w135:bool)
        n191 = flat-sequence {
          tunnel: w121 -> [w153]
          tunnel: [w150] -> w120
          frame #0 {
            n192 = control-ref of="Image (IMAQ)"() -> (w154:refnum<vi>)
            n193 = local read "Zoom old"() -> (w151:cluster{"X":sgl, "Y":sgl})
            n194 = local read "ratio(h)"() -> (w152:bool)
            n195 = call "updateZoom.vi"("Zoom old"=w151, "ratio(h)"=w152, "update Zoom"=w153, "imageRef"=w154) -> ("Zoom out"=w150:cluster{"X":sgl, "Y":sgl})  [unwired: 7 in]
          }
        }
        n196 = Select(t=w126, s=w123, f=w124) -> (s? t:f=w125:i32[])
        n197 = Or(x=w135, y=w121) -> (x .or. y?=w133:bool)
        n198 = And(x=w114, y=w133) -> (x .and. y?=w134:bool)
        n199 = case shown="True" w128 {
          tunnel: w146 -> [w223 _]
          tunnel: w143 -> [w220 w225]
          tunnel: [w222 w225] -> w142
          tunnel: w105 -> [w221 _]
          frame False {
            n200 = call "Update Indicators (Data String to ref array).vi"("Array"=w223, "Data String"=w221, "error in (no error)"=w220) -> ("error out"=w222:errorcluster)  [unwired: 11 in, 1 out]
          }
          frame True {
            n201 = Wait (ms)(milliseconds to wait=u32 100) -> ()  [unwired: 1 out]
          }
        }
        "error out" <- w142
        n202 = case shown="True" w106 {
          selector: w106 -> [_ w148]
          frame False {
          }
          frame True {
            n203 = call "StopFGV.vi"("Command"=enum16{"set", "get", "init"}."set", "Stop"=w148) -> ()  [unwired: 9 in, 1 out]
          }
        }
        n204 = case shown="True" w134 {
          tunnel: w120 -> [_ w207]
          tunnel: [w183 w207] -> w141
          tunnel: w140 -> [w183 _]
          tunnel: w115 -> [_ w208]
          tunnel: w136 -> [w182 _]
          tunnel: [w182 FALSE] -> w137
          tunnel: w113 -> [_ w192]
          tunnel: w112 -> [_ w188]
          tunnel: w122 -> [_ w185]
          frame False {
          }
          frame True {
            w189 = 0.0 ("lower limit")
            n205 = Multiply(x=w208, y=w207) -> (x*y=w206:cluster{sgl, sgl})
            n206 = control-ref of="Image (IMAQ)"() -> (w197:refnum<vi>)
            n207 = local read "fixsize"() -> (w198:bool)
            n208 = case shown="False" w198 {
              tunnel: w206 -> [w211 _]
              tunnel: w185 -> [w215 w219]
              tunnel: [w214 w219] -> w204
              tunnel: w197 -> [w213 _]
              frame False {
                n209 = property class="ImageControl"(reference=w213, "Image Area Size"=w211) -> ()  [unwired: 1 in, 2 out]
                n210 = Subtract(x=w211, y=cluster{sgl, sgl} {40.0, 70.0}) -> (x-y=w210:cluster{sgl, sgl})
                n211 = property on="Image (array)" class="IntGraph (strict)"("Plot Area Size"=w210) -> ()  [unwired: 2 in, 2 out]
                n212 = control-ref of="Pane"() -> (w216:refnum<vi>)
                n213 = control-ref of="Pane 4"() -> (w212:refnum<vi>)
                n214 = Unbundle(w211) -> (w217:sgl, w218:sgl)
                n215 = call "reSizeSplitter.vi"("this vi"=w215, "pane"=w216, "Width"=w217, "Height"=w218, "pane2"=w212) -> ("reference out"=w214:refnum<vi>)  [unwired: 10 in]
              }
              frame True {
              }
            }
            n216 = property on="Image (array)" class="IntGraph (strict)"() -> ("Plot Area Size"=w196:T10, "XScale.Minimum"=w190:dbl, "YScale.Minimum"=w187:dbl)  [unwired: 2 in, 2 out]
            n217 = property class="VI"(reference=w204) -> ("Front Panel.PanelBounds"=w203:T3)  [unwired: 1 in, 2 out]
            "old Panel Bounds" <- w203
            n218 = In Range and Coerce(upper limit=w192, x=w190, lower limit=w189) -> (coerced(x)=w191:dbl)  [unwired: 1 out]
            n219 = In Range and Coerce(upper limit=w188, x=w187, lower limit=w189) -> (coerced(x)=w186:dbl)  [unwired: 1 out]
            n220 = Unbundle By Name(w196) -> ("Width"=w195:u32, "Height"=w193:u32)
            n221 = Unbundle By Name(w203) -> ("right"=w202:i16, "left"=w201:i16)
            n222 = Subtract(x=w195, y=w191) -> (x-y=w194:dbl)
            n223 = Subtract(x=w193, y=w187) -> (x-y=w184:dbl)
            n224 = control-ref of="error message"() -> (w205:refnum<vi>)
            n225 = property on="Image (array)" class="IntGraph (strict)"("XScale.Minimum"=w191, "XScale.Maximum"=w194, "YScale.Minimum"=w186, "YScale.Maximum"=w184) -> ()  [unwired: 2 in, 2 out]
            n226 = Subtract(x=w202, y=w201) -> (x-y=w200:i16)
            n227 = property class="Str"(reference=w205, "Width"=w200) -> ()  [unwired: 1 in, 2 out]
          }
        }
        n228 = control-ref of="error (h)"() -> (w111:refnum<vi>)
        n229 = control-ref of="error message"() -> (w130:refnum<vi>)
        n230 = call "clearErrorMessageGUI.vi"("millisecond timer value"=w131, "Boolean"=w128, "error message"=w130, "reference"=w111) -> ("millisecond timer value 2"=w132:u32)
        n231 = call "StatusDataConnectionFGV.vi"("Command"=enum16{"get", "set", "init"}."get") -> ("Data Connection out"=→"image connection":bool)  [unwired: 10 in]
        n232 = call "StatusImageConnectionFGV.vi"("Command"=enum16{"get", "set", "init"}."get") -> ("Image Connection out"=→"data connection ok":bool)  [unwired: 10 in]
        "Image (IMAQ)" <- w116
      }
      n233 = local read "connections (hidden)"() -> (w93:variant[])
      n234 = call "IMAQ Dispose"("Image"=w101) -> ()  [unwired: 5 in, 1 out]
      n235 = call "Close UDP AND TCP connections.vi"("error in"=w98, "appended array"=w93) -> ()  [unwired: 6 in]
    }
    frame #3 {
      n236 = flat-sequence {
        frame #0 {
          n237 = Wait (ms)(milliseconds to wait=u32 0) -> ()  [unwired: 1 out]
        }
        frame #1 {
          n238 = local write "stop"(FALSE ("stop")) -> ()
        }
        frame #2 {
          n239 = control-ref of="This VI"() -> (w348:refnum<vi>)
          n240 = case shown="True" FALSE {
            tunnel: w348 -> [w349 w352]
            tunnel: [w349 w350] -> w347
            frame False {
            }
            frame True {
              n241 = property class="VI" props=["Front Panel.Open"](reference=w352) -> (reference out=w351:refnum<vi>)  [unwired: 1 in, 2 out]
              n242 = invoke class="VI" method="FP.Close"(reference=w351) -> (reference out=w350:refnum<vi>)  [unwired: 2 in, 2 out]
            }
          }
          n243 = Close Reference(reference=w347) -> ()  [unwired: 1 in, 1 out]
        }
      }
      n244 = control-ref of="Main  Control"() -> (w342:refnum<vi>)
      n245 = property class="TabCtl (strict)"(reference=w342, "Tabs Visible?"=TRUE) -> ()  [unwired: 1 in, 2 out]
      n246 = property class="TabCtl (strict)"(reference=w342, "Tab Location"=enum32{"Top", "Bottom", "Left", "Right"}."Bottom") -> ()  [unwired: 1 in, 2 out]
    }
  }
